vi "repeated_capability_parameters.vi"(2 "error in":errorcluster, 3 "Instrument Command In":string) -> (0 "error out":errorcluster, 1 "Instrument Command Out":string)   [LabVIEW 2018]
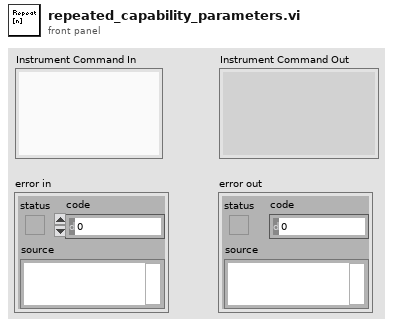
[diagram p1: front panel]
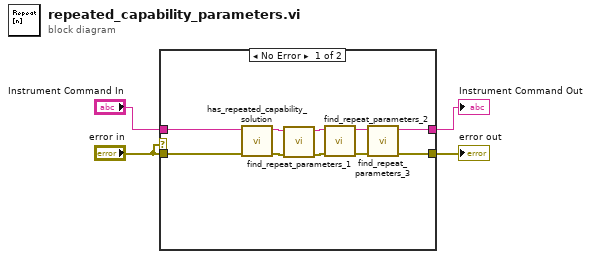
[diagram p0: block diagram]
diagram:
  n1 = case shown="No Error" "error in" {
    tunnel: [w14 w15] -> w4
    tunnel: [w13 w16] -> w3
    tunnel: "error in" -> [w5 w15]
    tunnel: "Instrument Command In" -> [w6 w16]
    frame No Error {
      n2 = call "has_repeated_capability_solution.vi"("error in (no error)"=w5, "Instrument Command In"=w6) -> ("error out"=w12:errorcluster, "Instrument Command Out"=w11:string)  [unwired: 8 out]
      n3 = call "find_repeat_parameters_1.vi"("error in (no error)"=w12, "String In"=w11) -> ("error out"=w7:errorcluster, "String Out"=w8:string)  [unwired: 8 out]
      n4 = call "find_repeat_parameters_2.vi"("error in (no error)"=w7, "String In"=w8) -> ("error out"=w10:errorcluster, "String Out"=w9:string)  [unwired: 8 out]
      n5 = call "find_repeat_parameters_3.vi"("error in (no error)"=w10, "String In"=w9) -> ("error out"=w14:errorcluster, "String Out"=w13:string)  [unwired: 8 out]
    }
    frame Error {
    }
  }
  "error out" <- w4
  "Instrument Command Out" <- w3
